vi "LaserController.vi"(5 "Laser Pin":u8, 7 "Trigger Pin":u8, 8 "Error In":errorcluster, 9 "Energy In":dbl, 10 "Overheat In":bool, 11 "LINX Resource In":T1) -> (0 "Error Out":errorcluster, 1 "Energy Out":dbl, 2 "Overheat Out":bool, 3 "LINX Resource Out":T1)   [LabVIEW 2022 SP3]
uses:
  <vilib>/MakerHub/LINX/Private/Type Defs/LINX Ref.ctl
  <vilib>/MakerHub/LINX/Private/Type Defs/Platform.ctl
  <vilib>/MakerHub/LINX/Private/Type Defs/Interface.ctl
  <vilib>/MakerHub/LINX/Private/Device/Type Defs/LINX Device Config.ctl
  <vilib>/MakerHub/LINX/Private/Device/Type Defs/TCP Config.ctl
  <vilib>/MakerHub/LINX/Private/Device/Type Defs/Channels.ctl
  <vilib>/MakerHub/LINX/Public/Peripherals/Digital/Digital Read 1 Chan.vi
  <vilib>/MakerHub/LINX/Public/Peripherals/PWM/PWM Set Duty Cycle 1 Chan.vi
  <vilib>/MakerHub/LINX/Public/Peripherals/Digital/Digital Read N Chans.vi
  <vilib>/MakerHub/LINX/Private/Local IO/LinxDigitalRead.vi
  <vilib>/MakerHub/LINX/Public/Utilities/Check Channel.vi
  <vilib>/MakerHub/LINX/Private/Utilties/Generate Error.vi
  <vilib>/MakerHub/LINX/Public/Peripherals/PWM/PWM Set Duty Cycle N Chans.vi
  <vilib>/MakerHub/LINX/LMH-LINX.lvlib
  <vilib>/MakerHub/LINX/Private/Device/Device.lvlib
panel:
  out "DI Value":bool
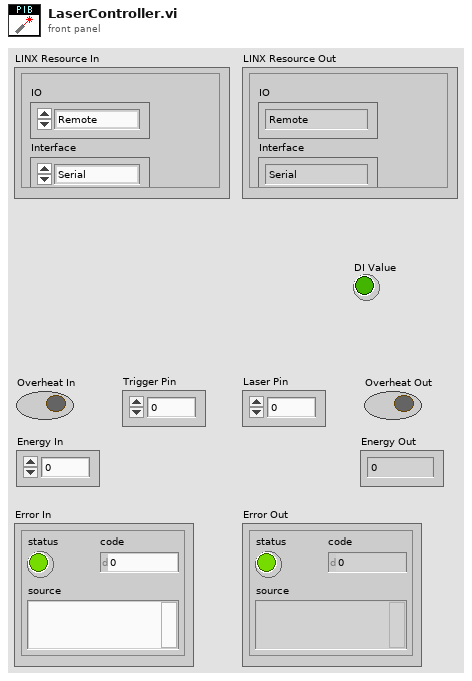
[diagram p1: front panel]
types:
  T1 = typedef "LMH-LINX.lvlib/LINX Ref.ctl" = cluster{"IO":T2, "Interface":T3, "LINX Device Config":T4}
  T2 = typedef "LMH-LINX.lvlib/Platform.ctl" = enum16{"Remote", "Local"}
  T3 = typedef "LMH-LINX.lvlib/Interface.ctl" = enum16{"Serial", "TCP"}
  T4 = typedef "LMH-LINX.lvlib/Device.lvlib/LINX Device Config.ctl" = cluster{"Interface":T3, "COM Port":refnum<visa-resource-name>, "TCP Configuration":T5, "Device Family":u8, "Device ID":u8, "Device Name":string, "TCP Ref":refnum<k5>, "Channels":T6}
  T5 = typedef "LMH-LINX.lvlib/Device.lvlib/TCP Config.ctl" = cluster{"IP Address":string, "Port":u16}
  T6 = typedef "LMH-LINX.lvlib/Channels.ctl" = cluster{"DI":u8[], "DO":u8[], "AI":u8[], "AO":u8[], "PWM":u8[], "QE":u8[], "UART":u8[], "I2C 2":u8[], "SPI":u8[], "CAN":u8[], "Servo":u8[], "AI Ref (V)":dbl, "AI Resolution (Bits)":u8, "AO Ref (V)":dbl, "AO Resolution (Bits)":u8}
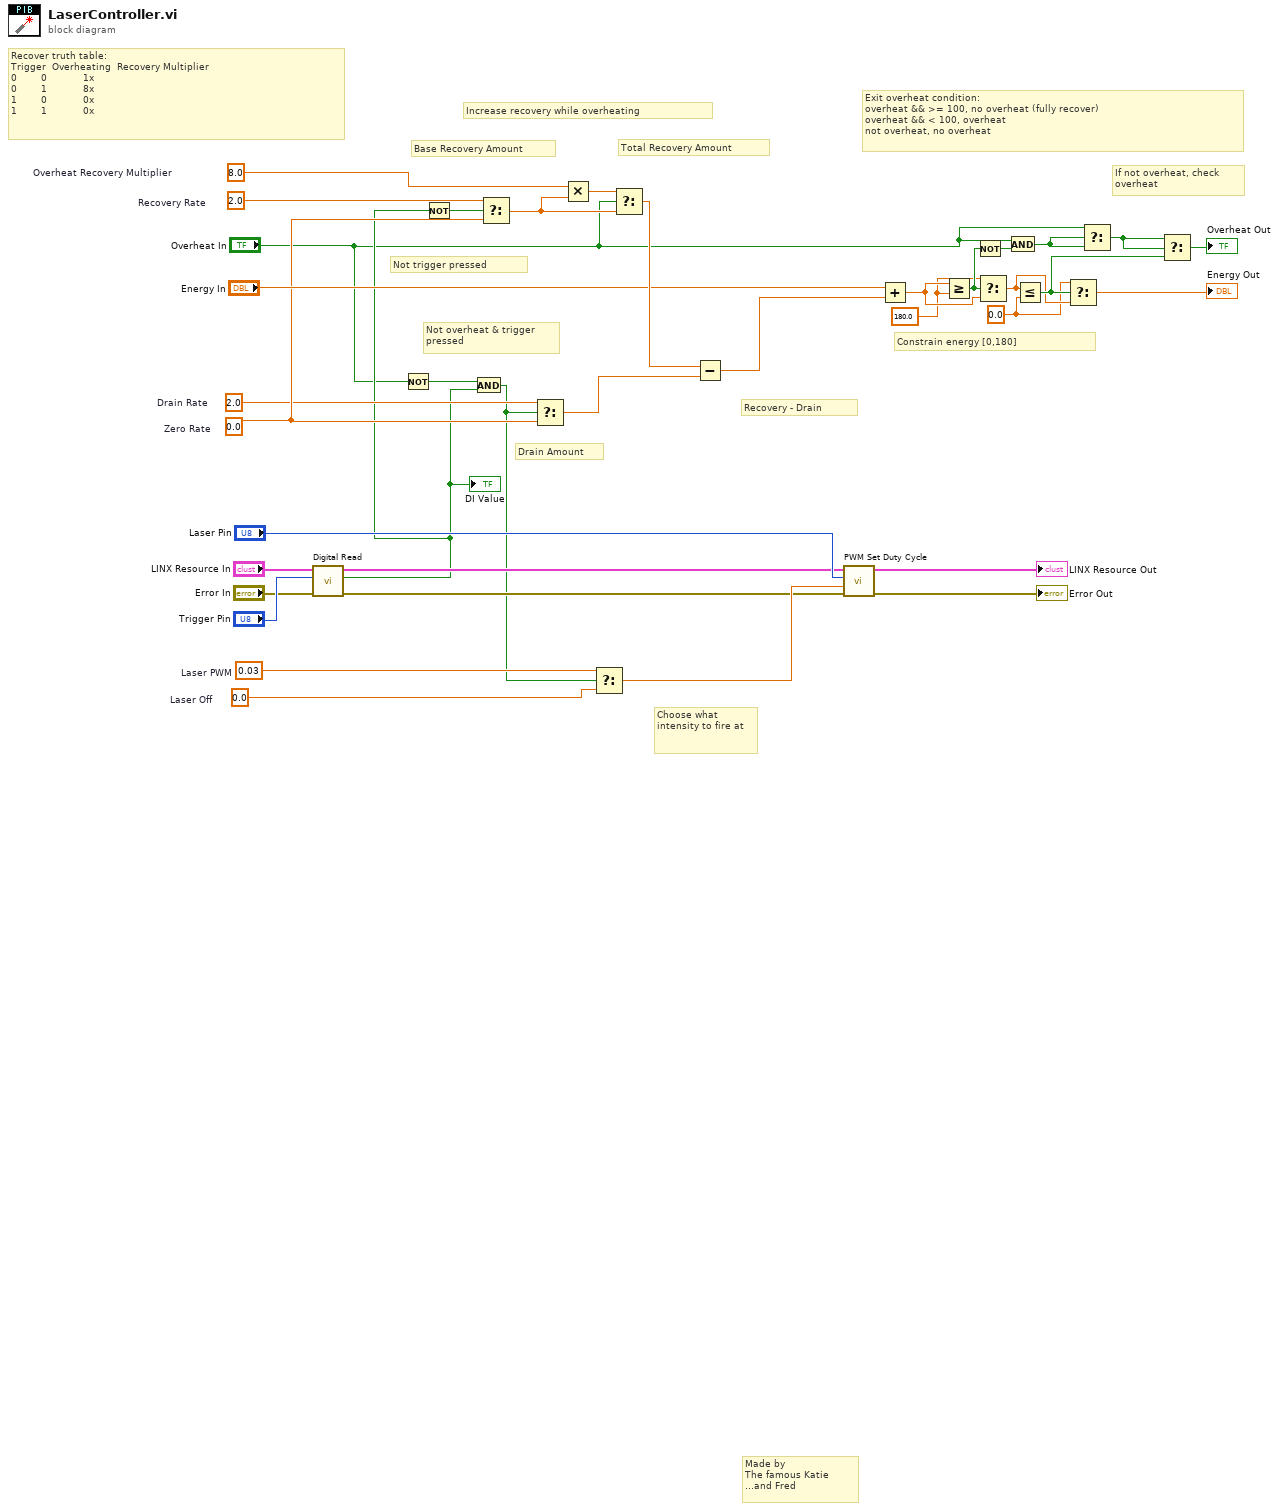
[diagram p0: block diagram]
diagram:
  w5 = 0.03  # Laser PWM
  w6 = 2.0  # Recovery Rate
  w7 = 2.0  # Drain Rate
  w3 = 8.0  # Overheat Recovery Multiplier
  w24 = 0.0 ("y")
  w21 = 180.0 ("y")
  w17 = 0.0  # Laser Off
  w14 = 0.0  # Zero Rate
  # "Made by\nThe famous Katie\n...and Fred"
  # "Not trigger pressed"
  # "Base Recovery Amount"
  # "Not overheat & trigger pressed"
  # "Drain Amount"
  # "Total Recovery Amount"
  # "Recovery - Drain"
  # "Recover truth table:\nTrigger  Overheating  Recovery Multiplier\n0        0            1x\n0        1            8x\n1        0            0x\n1        1            0x"
  # "Increase recovery while overheating"
  # "If not overheat, check overheat"
  # "Exit overheat condition:\noverheat && >= 100, no overheat (fully recover)\noverheat && < 100, overheat\nnot overheat, no overheat"
  # "Choose what intensity to fire at"
  # "Constrain energy [0,180]"
  n1 = call-poly <vilib>:"Digital Read.vi"("Error In"="Error In", "DI Channel"="Trigger Pin", "LINX Resource"="LINX Resource In") -> ("Error Out"=w10:errorcluster, "DI Value"=w4:bool, "LINX Resource"=w11:T1)  [unwired: 6 in]
  "DI Value" <- w4
  n2 = Not(x="Overheat In") -> (.not. x?=w33:bool)
  n3 = Not(x=w4) -> (.not. x?=w37:bool)
  n4 = And(x=w33, y=w4) -> (x .and. y?=w2:bool)
  n5 = Select(t=w6, s=w37, f=w14) -> (s? t:f=w36:dbl)
  n6 = Select(t=w7, s=w2, f=w14) -> (s? t:f=w19:dbl)
  n7 = Multiply(x=w3, y=w36) -> (x*y=w35:dbl)
  n8 = Select(t=w5, s=w2, f=w17) -> (s? t:f=w18:dbl)
  n9 = Select(t=w35, s="Overheat In", f=w36) -> (s? t:f=w34:dbl)
  n10 = Subtract(x=w34, y=w19) -> (x-y=w20:dbl)
  n11 = call-poly <vilib>:"PWM Set Duty Cycle.vi"("Error In"=w10, "Duty Cycle (0-1)"=w18, "PWM Channel"="Laser Pin", "LINX Resource"=w11) -> ("Error Out"=→"Error Out":errorcluster, "LINX Resource"=→"LINX Resource Out":T1)  [unwired: 6 in]
  n12 = Add(x="Energy In", y=w20) -> (x+y=w22:dbl)
  n13 = Greater Or Equal?(x=w22, y=w21) -> (x >= y?=w29:bool)
  n14 = Not(x=w29) -> (.not. x?=w30:bool)
  n15 = Select(t=w21, s=w29, f=w22) -> (s? t:f=w25:dbl)
  n16 = And(x="Overheat In", y=w30) -> (x .and. y?=w32:bool)
  n17 = Less Or Equal?(x=w25, y=w24) -> (x <= y?=w27:bool)
  n18 = Select(t=w24, s=w27, f=w25) -> (s? t:f=→"Energy Out":dbl)
  n19 = Select(t="Overheat In", s=w32, f=w32) -> (s? t:f=w31:bool)
  n20 = Select(t=w31, s=w31, f=w27) -> (s? t:f=→"Overheat Out":bool)
